vi "module2.vi"(11 "controlName2":i16) -> (3 "indicatorName2":i16)   [LabVIEW 2021]
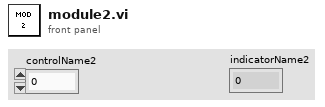
[diagram p1: front panel]
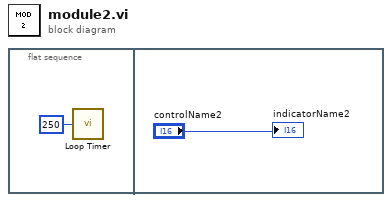
[diagram p0: block diagram]
diagram:
  n1 = flat-sequence {
    frame #0 {
      n2 = call "Loop Timer"("Count(mSec)"=u32 250) -> ()  [unwired: 1 out]
    }
    frame #1 {
      "indicatorName2" <- "controlName2"
    }
  }
